vi "Dashboard Main.vi"() -> ()   [LabVIEW 2016]
uses:
  <vilib>/Utility/miscctls.llb/LVRowAndColumnTypeDef.ctl
  <vilib>/event_ctls.llb/eventvkey.ctl
  <vilib>/Rock Robotics/Network Tables/NT Read Numeric Array.vi
  <vilib>/Rock Robotics/Network Tables/NT Write Numeric Array.vi
  <vilib>/Rock Robotics/WPI/Dashboard/WPI_DashboardLogging Global.vi
panel:
  in  "Camera Settings Right":T1={"Frame Rate"=30, "Compression"=30, "Size"=1, "DB Camera Config"=FALSE} {"Frame Rate" scale=1.0..30.0; "Compression" scale=100.0..-1.0; "Size" items=["640x480", "320x240", "160x120"]}
  in  "Camera Name Right":string(combo)="No Camera Selection"
  out "Camera Info":cluster{"Mbps LED":bool, "Mbps":dbl, "fps":dbl} {"fps" format="%#.1g"; "Mbps" format="%#.1g"}
  in  "Camera Settings":T1={"Frame Rate"=30, "Compression"=30, "Size"=1, "DB Camera Config"=FALSE} {"Frame Rate" scale=1.0..30.0; "Compression" scale=100.0..-1.0; "Size" items=["640x480", "320x240", "160x120"]}
  in  "TCP":refnum<k5>
  in  "Rec Mode":enum32{"Stop", "Record", "Playback"}(radio)
  out "Robot IP":string
  out "Image Message":string="Timeout in Camera Communications"
  in  "Dashboard Tab":T2(tab)
  in  "Select Auto":string(combo)="Select Autonomous ..."
  out "NT Connection":bool
  out "MotorChart R":cluster{"Numeric":dbl, "Numeric":dbl}(graph)
  out "MotorChart L":cluster{"Numeric":dbl, "Numeric":dbl}(graph)
  out "MotorSliders R":cluster{"MotorSlide1":dbl, "MotorSlide2":dbl} {"MotorSlide2" scale=-1.0..1.0 scale format="%#_2e"; "MotorSlide1" scale=-1.0..1.0 scale format="%#_2e"}
  out "MotorSliders L":cluster{"MotorSlide1":dbl, "MotorSlide2":dbl} {"MotorSlide2" scale=-1.0..1.0 scale format="%#_2e"; "MotorSlide1" scale=-1.0..1.0 scale format="%#_2e"}
  out "Gyro":dbl(knob) scale=0.0..360.0
  out "JS1 Z":dbl(slide) scale=-1.0..1.0 scale format="%#_2e"
  out "JS1 Graph":cluster{"X":dbl, "Y":dbl}[](graph)
  out "JS1 Buttons":T3
  out "JS2 Z":dbl(slide) scale=-1.0..1.0 scale format="%#_2e"
  out "JS2 Graph":cluster{"X":dbl, "Y":dbl}[](graph)
  out "JS2 Buttons":T3
  out "Mode":T4(ring)=enum."Auto Disabled"
  out "Camera Image Right":T5(plugin-control)
  out "Left Encoder":dbl
  out "Right Encoder":dbl
  in  "Save":bool
  in  "Teleop Controls":T6(tab)
  in  "Y Axis":T7
  in  "X Axis":T7
  in  "Forward Trim":T8={"Trim Max"=0.37, "Trim Min"=0.01, "Trim Deadzone"=0.1, "Trim LR"=TRUE}
  in  "Backward Trim":T8={"Trim Max"=0.5, "Trim Min"=0.05, "Trim Deadzone"=0.1, "Trim LR"=FALSE}
  in  "PID Tuning":enum32{"Drive with PID", "Turn by Angle"}(tab)
  in  "Drive with PID":T9={"Max Speed"=0.7, "P/I/D"=[1.0, 0.0, 0.01], "Min Speed"=0.4, "Accel Distance"=64.0}
  in  "Turn By Angle":T10={"P/I/D"=[0.25, 0.001, 0.0], "Turn Speed"=0.55, "Linearity"=0.6}
  in  "Autonomous Distances":T11(tab)
  in  "Station 1 Angle":dbl=60.0
  in  "Station 1":dbl[](array[numeric])=[97.0, 30.0, -30.0, 120.0]
  in  "Station 2":dbl[](array[numeric])=[82.0, -48.0, 48.0, 120.0]
  in  "Station 3 Angle":dbl=-60.0
  in  "Station 3":dbl[](array[numeric])=[96.0, 30.0, -30.0, 120.0]
  in  "Drive Forward":dbl[](array[numeric])=[82.0, 0.0, 0.0, 0.0]
  in  "Gear and B":dbl[](array[numeric])=[82.0, -48.0, 0.0, 0.0]
  in  "Test Slider":dbl(slide) scale=0.0..100.0 scale format="%#_3g"
  in  "On/Off":bool caption="Solenoid"
  in  "Test Name":u16(ring) items=["Select the test to run..."]
  in  "Test Tree":string(tree)
  in  "Motor":cluster{"Value":dbl, "Enable":bool} {"Value" scale=-1.0..1.0 scale format="%#_3g"}
  out "Progress":T12 {"Test Progress" scale=0.0..100.0}
  in  "Rev/Fwd":cluster{"Forward":bool, "Reverse":bool}
  in  "Test Ring":u16(ring) items=["Monochrome", "Color"]
  out "Cmd Status":string
  in  "Execute Command":bool
  in  "Command Params":string[][](table)
  in  "Command Selection":i32(listbox)
  in  "CheckList":i32(listbox)
  out "Tree":string(tree)
  out "Camera Image":T5(plugin-control)
  in  "Camera Name":string(combo)="No Camera Selection"
  out "Background":bool
  # "HW"
  # "HW"
  # "Joysticks"
  # "Drive Motors"
  # "Front"
  # "Right"
  # "Left"
  # "Back"
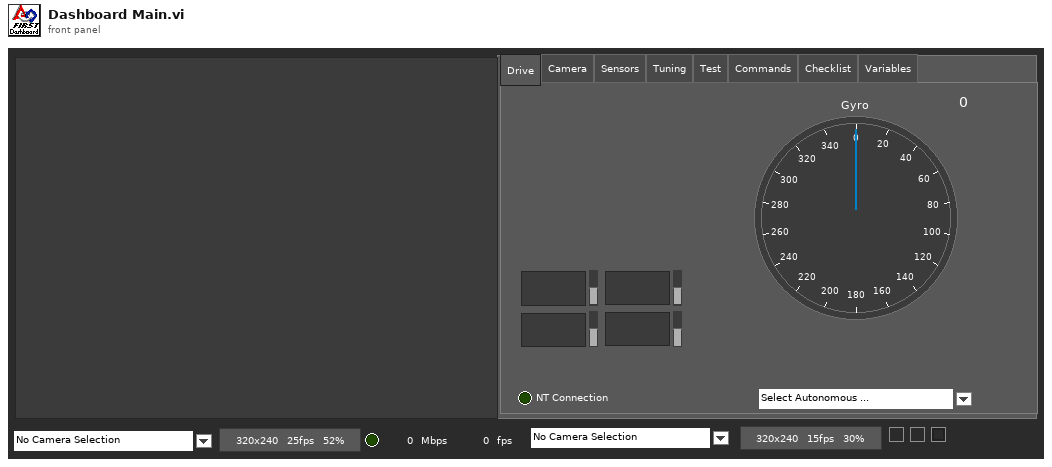
[diagram p1: front panel]
types:
  T1 = cluster{"Frame Rate":i32, "Compression":i32, "Size":u16, "DB Camera Config":bool}
  T2 = enum32{"Drive", "Camera", "Sensors", "Tuning", "Test", "Commands", "Checklist", "Variables"}
  T3 = cluster{bool, bool, bool, bool, bool, bool, bool, bool, bool, bool, bool, bool}
  T4 = enum8{"Tele-Op Disabled", "Tele-Op Enabled", "Auto Disabled", "Auto Enabled", "Test Disabled", "Test Enabled", "Disconnected", "No Code", "E-Stop"}
  T5 = typedef "IMAQ Image.ctl" = refnum<image>
  T6 = enum32{"Speed Sensitivity", "Turn Sensitivity", "Forward Trim", "Backwards Trim"}
  T7 = cluster{"Max Speed":dbl, "Min Speed":dbl, "Deadzone":dbl}
  T8 = cluster{"Trim Max":dbl, "Trim Min":dbl, "Trim Deadzone":dbl, "Trim LR":bool}
  T9 = cluster{"Max Speed":dbl, "P/I/D":dbl[], "Min Speed":dbl, "Accel Distance":dbl}
  T10 = cluster{"P/I/D":dbl[], "Turn Speed":dbl, "Linearity":dbl}
  T11 = enum32{"Station 1", "Station 2", "Station 3", "Drive Forward", "Gear and Back"}
  T12 = cluster{"Test Progress":u8, "Test Progress Text":string}
  T13 = typedef "Image Type" = u32
  T14 = cluster{"IDs":cluster{"RPC field ID":u16, "Unique ID":u16}, "String":string}
  T15 = enum32{"Drive", "Basic", "Custom", "Test", "Checklist", "Variables"}
  T16 = cluster{"Error Strings":string, "Disable Counts":cluster{u16, u16}, "Rail Faults":cluster{u16, u16, u16}, "Robot IP":string, "DB Mode":u8, "Event Info":cluster{"Name":string, "Type":u8, "Number":u16, "Replay":u8}}
  T17 = cluster{"Storage":cluster{"Disk Free":u64, "RAM Block":u32, "RAM free":u32}, "CPU Utilization":cluster{"CPU % ISR":sgl, "CPU % Time Crit":sgl, "CPU % Timed Str":sgl, "CPU % High":sgl, "CPU % Above":sgl, "CPU % Normal":sgl, "CPU % Low":sgl}, "CAN":cluster{"% Bus Utilization":sgl, "Bus Off Cnt":u32, "TX_FIFO Full Cnt":u32, "Receive Error Cnt":u8, "Transmit Error Cnt":u8}, "HID":cluster{"HID Outputs":u32, "Rumble Low":u16, "Rumble High":u16}[]}
  T18 = cluster{"Status bits":cluster{"Test Mode":bool, "Autonomous":bool, "Enabled":bool, "Code Start":bool, "Brownout":bool, "Reserved 2":bool, "Reserved 3":bool, "E-Stop":bool}, "Code Trace":cluster{"Disabled":bool, "TeleOp":bool, "Auto":bool, "Test":bool}, "Controller Type":enum16{"unknown", "cRIO", "roboRio"}, "Code?":enum16{"unknown", "noCode", "code"}, "Battery V":dbl}
  T19 = cluster{"Control Bits":cluster{"TestMode":bool, "Autonomous":bool, "Enabled":bool, "FMS Present":bool, bool, bool, bool, "E-Stop":bool}, "Team Station ":u8, "Countdown":sgl, "Joystick Values":cluster{"Axes":dbl[], "Buttons":bool[], "POVs":i16[]}[]}
  T20 = cluster{"Axes":dbl[], "Buttons":bool[], "POVs":i16[]}[]
  T21 = cluster{"Axes":dbl[], "Buttons":bool[], "POVs":i16[]}
  T22 = cluster{"Buttons[0]":bool, "Buttons[1]":bool, "Buttons[2]":bool, "Buttons[3]":bool, "Buttons[4]":bool, "Buttons[5]":bool, "Buttons[6]":bool, "Buttons[7]":bool, "Buttons[8]":bool, "Buttons[9]":bool, "Buttons[10]":bool, "Buttons[11]":bool}
  T23 = cluster{"X Axis":cluster{"Max Speed":dbl, "Min Speed":dbl, "Deadzone":dbl}, "Y Axis":cluster{"Max Speed":dbl, "Min Speed":dbl, "Deadzone":dbl}, "Forward Trim":cluster{"Trim Max":dbl, "Trim Min":dbl, "Trim Deadzone":dbl, "Trim LR":bool}, "Backward Trim":cluster{"Trim Max":dbl, "Trim Min":dbl, "Trim Deadzone":dbl, "Trim LR":bool}, "Drive with PID":cluster{"Max Speed":dbl, "P/I/D":dbl[], "Min Speed":dbl, "Accel Distance":dbl}, "Turn By Angle":cluster{"P/I/D":dbl[], "Turn Speed":dbl, "Linearity":dbl}}
  T24 = cluster{"Camera Image":refnum<vi>, "Dashboard Tab":refnum<vi>, "Background":refnum<vi>, "Rec Mode":refnum<vi>, "Test Slider":refnum<vi>, "On/Off ":refnum<vi>, "Test Ring":refnum<vi>, "Rev/Fwd":refnum<vi>, "Test Name":refnum<vi>, "Motor":refnum<vi>, "Progress":refnum<vi>, "CheckList":refnum<vi>, "Tree":refnum<vi>, "Test Tree":refnum<vi>, "Command Params":refnum<vi>, "Command Selection":refnum<vi>, "Execute Command":refnum<vi>, "Cmd Status":refnum<vi>, "Camera Settings":refnum<vi>, "Camera Name":refnum<vi>, "Camera Info":refnum<vi>, "Camera Settings Right":refnum<vi>, "Camera Name Right":refnum<vi>, "Camera Image Right":refnum<vi>}
  T25 = cluster{"Operation":enum16{"Update", "Clear"}, "Color Box":u32}[]
  T26 = typedef "eventvkey.ctl" = enum16{"ASCII", "Enter", "Return", "Shift", "Ctrl", "Alt", "Cmd", "Opt", "Caps", "NumLock", "Clear", "Break", "Up", "Down", "Left", "Right", "Insert", "Delete", "Home", "End", "PageUp", "PageDown", "Escape", "Help", "Pause", "ScrollLock", "F1", "F2", "F3", "F4", "F5", "F6", "F7", "F8", "F9", "F10", "F11", "F12", "F13", "F14", "F15", "F16", "F17", "F18", "F19", "F20", "F21", "F22", "F23", "F24", "Play", "VolumeUp", "VolumeDown", "Mute", "Two Byte Char"}
  T27 = cluster{"Image Size":bool, "Image Type":bool, "Pixel Value":bool, "ROI Information":bool, "Zoom Factor":bool}
  T28 = cluster{"Operation":enum16{"Update", "Clear"}, "Color Box":u32}
  T29 = typedef "LVRowAndColumnTypeDef.ctl" = cluster{"Row":i32, "Column":i32}
  T30 = cluster{"Shift":bool, "Ctrl":bool, "Alt":bool, "Cmd":bool, "Opt":bool}
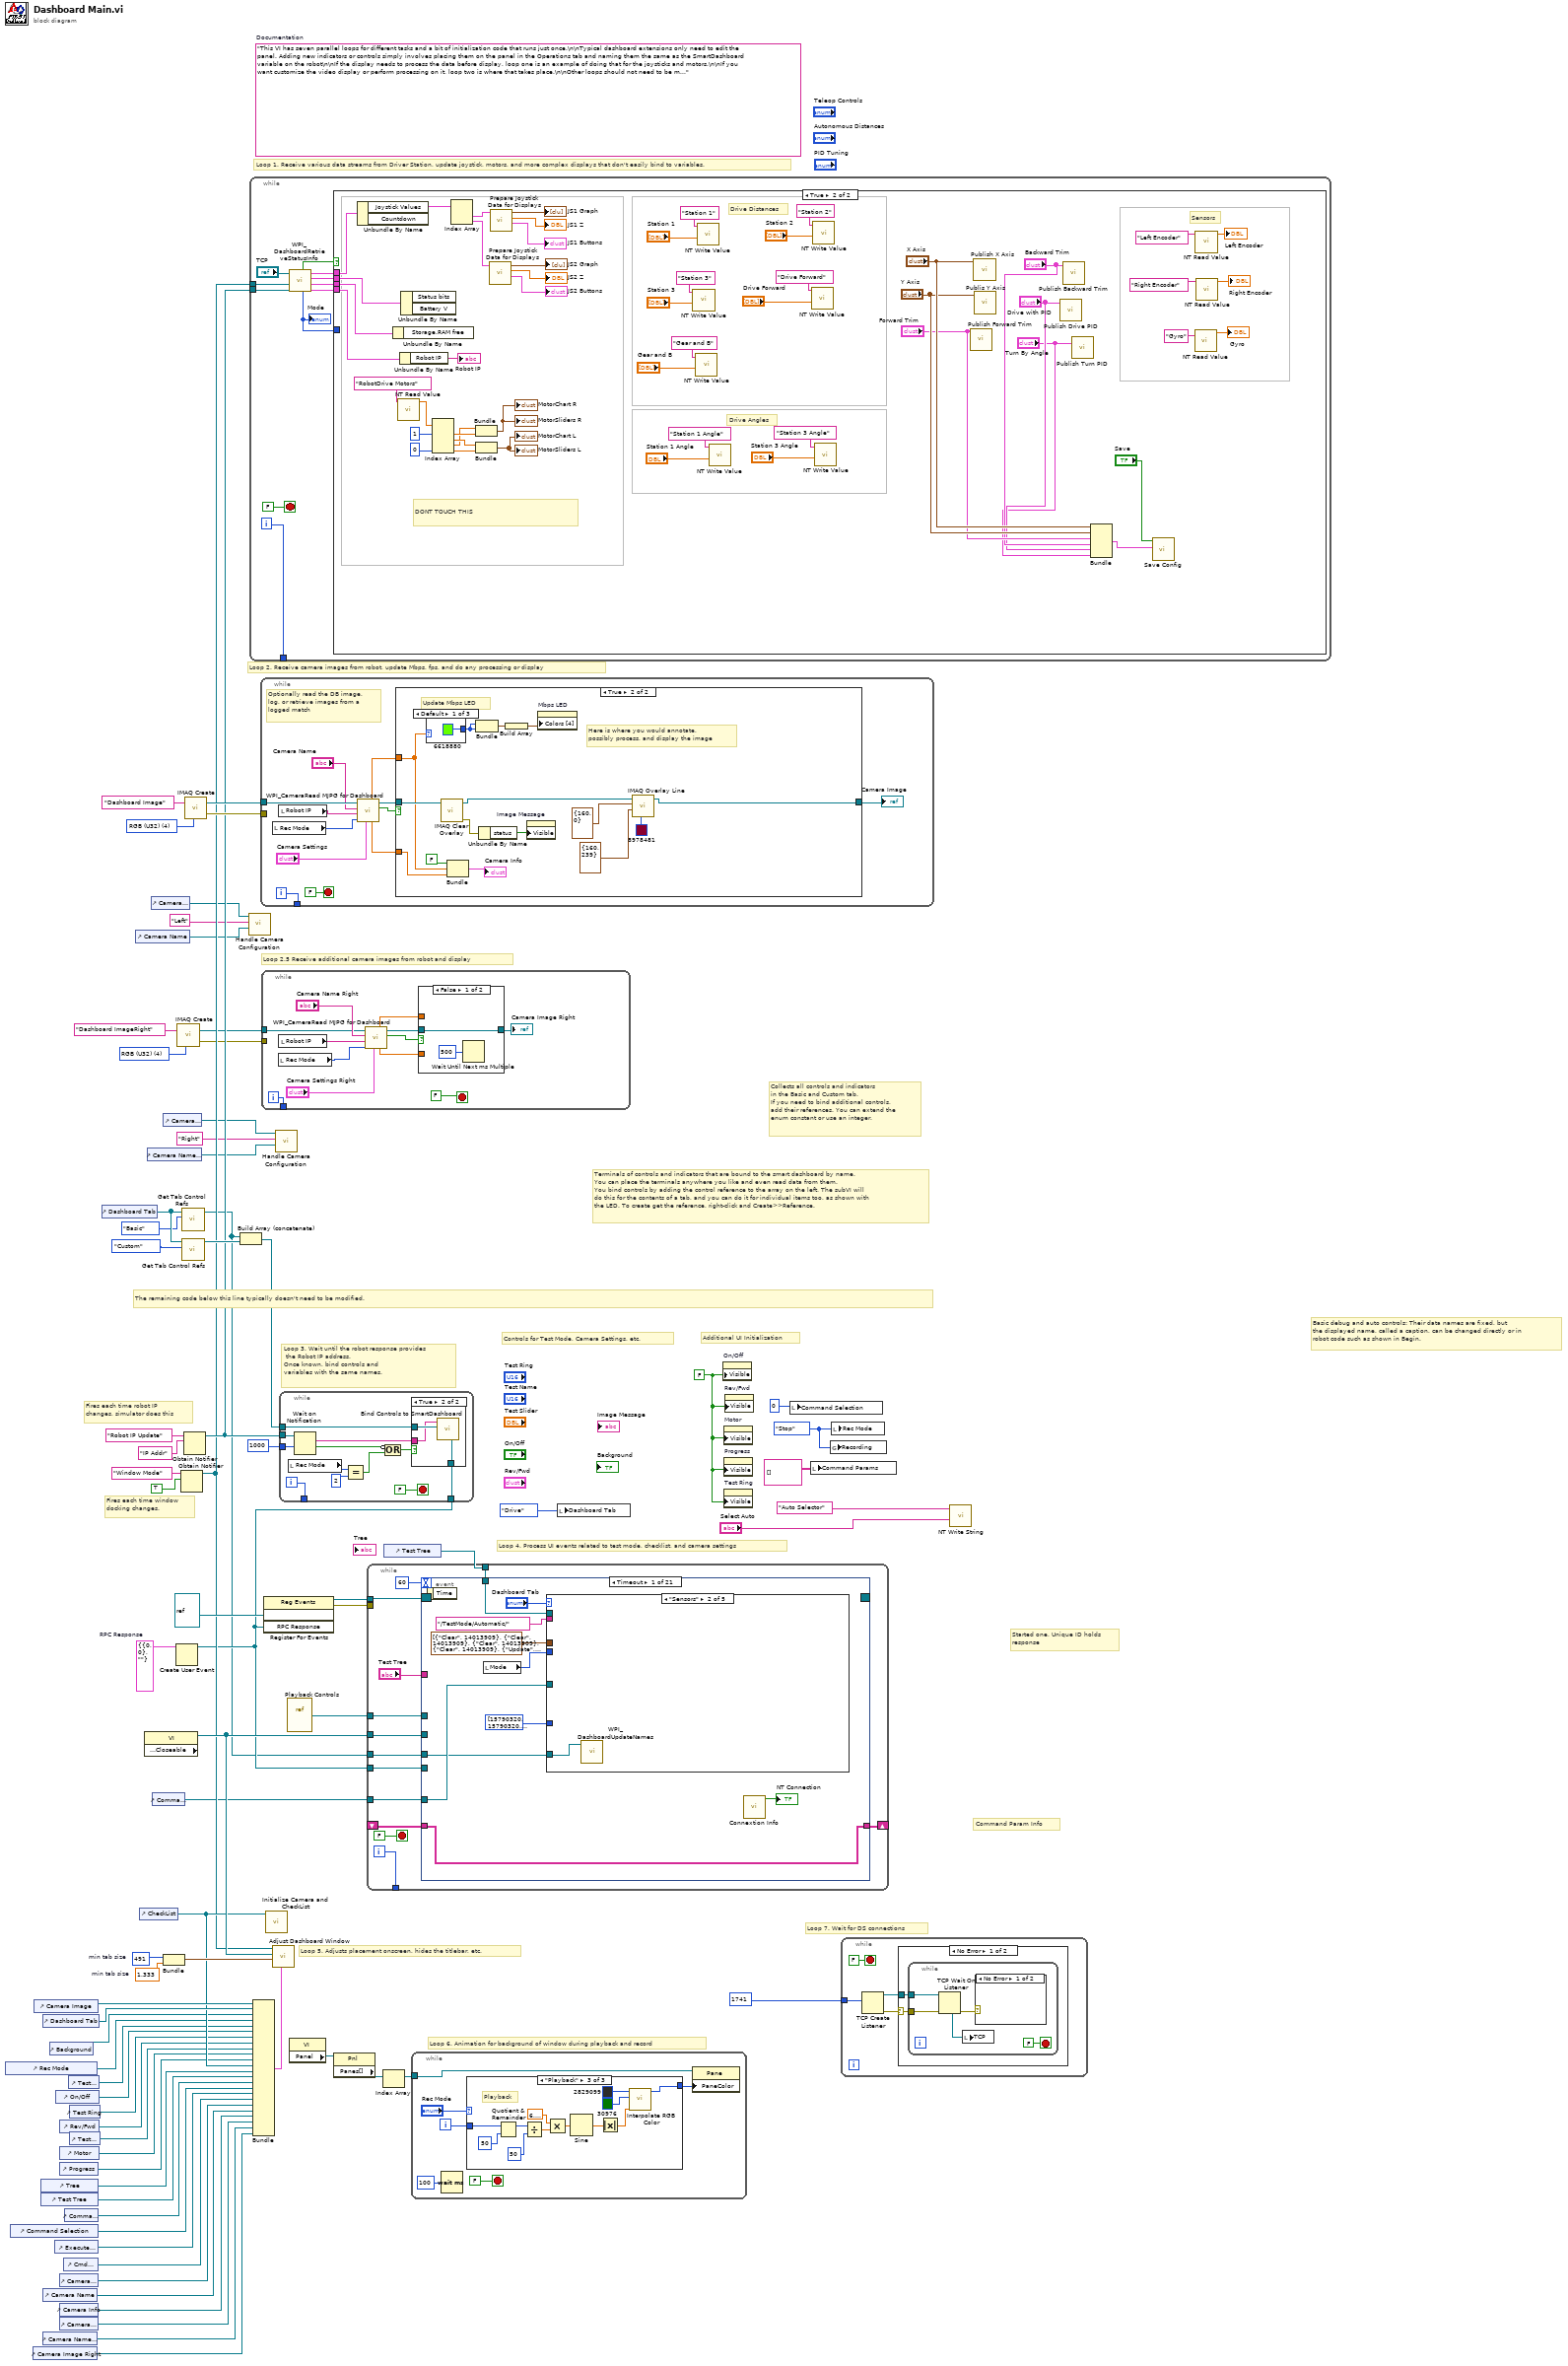
[diagram p0: block diagram]
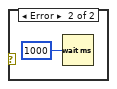
[diagram p3: hidden frame]
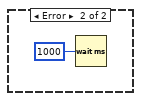
[diagram p4: hidden frame]
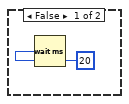
[diagram p5: hidden frame]
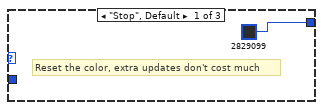
[diagram p6: hidden frame]
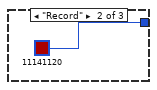
[diagram p7: hidden frame]
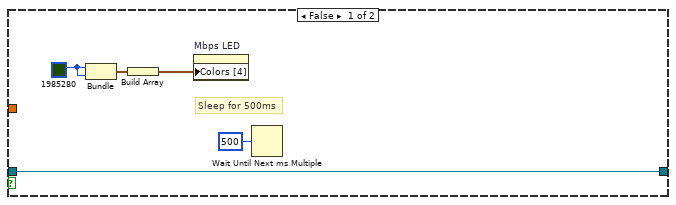
[diagram p9: hidden frame]
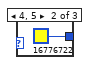
[diagram p10: hidden frame]
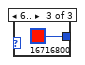
[diagram p11: hidden frame]
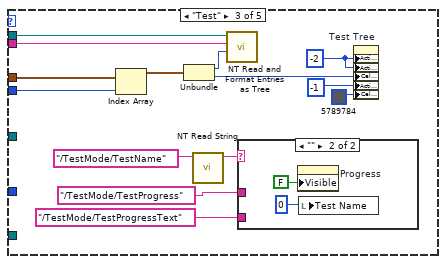
[diagram p13: hidden frame]
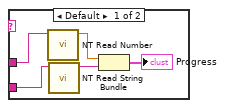
[diagram p14: hidden frame]
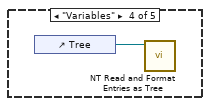
[diagram p15: hidden frame]
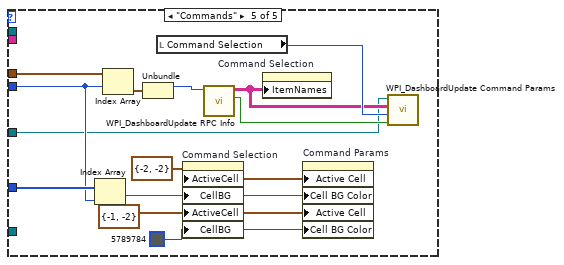
[diagram p16: hidden frame]
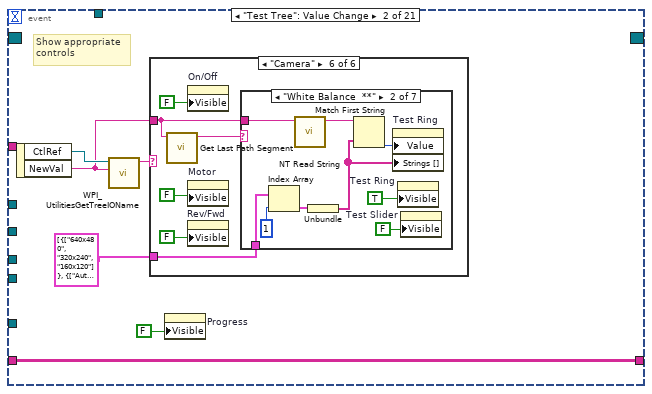
[diagram p17: hidden frame]
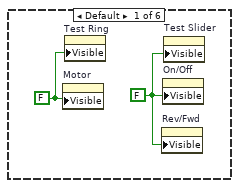
[diagram p18: hidden frame]
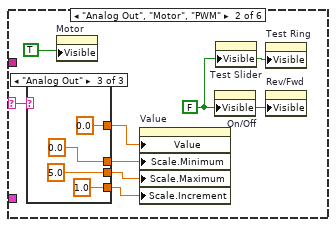
[diagram p19: hidden frame]
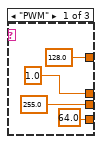
[diagram p20: hidden frame]
diagram:
  w11 = T13 4 items=["Grayscale (U8)", "Grayscale (I16)", "Grayscale (SGL)", "Complex (CSG)", "RGB (U32)", "HSL (U32)", "RGB (U64)"] ("Image Type")
  w27 = T14 {"IDs"={"RPC field ID"=0, "Unique ID"=0}, "String"=""}  # RPC Response
  w51 = 491  # min tab size
  w50 = 1.333  # min tab size
  w58 = enum32{"Stop", "Record", "Playback"}."Stop" ("Rec Mode")
  w34 = FALSE ("Visible")
  (unwired) "This VI has seven parallel loops for different tasks and a bit of initialization code that runs just once.\n\nTypical dashboard extensions only need to edit the panel. Adding new indicators or controls simply involves placing them on the panel in the Operations tab and naming them the same as the SmartDashboard variable on the robot\n\nIf the display needs to process the data before display, loop one is an example of doing that for the joysticks and motors.\n\nIf you want customize the video display or perform processing on it, loop two is where that takes place.\n\nOther loops should not need to be modified. They are pretty standard, and document the task they perform."  # Documentation
  w75 = T13 4 items=["Grayscale (U8)", "Grayscale (I16)", "Grayscale (SGL)", "Complex (CSG)", "RGB (U32)", "HSL (U32)", "RGB (U64)"] ("Image Type")
  # "Loop 2.5 Receive additional camera images from robot and display"
  # "Command Param Info"
  # "Started one, Unique ID holds\nresponse"
  # "Loop 7. Wait for DS connections"
  # "Basic debug and auto controls: Their data names are fixed, but\nthe displayed name, called a caption, can be changed directly or in\nrobot code such as shown in Begin."
  # "Controls for Test Mode, Camera Settings, etc."
  # "Additional UI Initialization"
  # "Loop 6. Animation for background of window during playback and record"
  # "Fires each time robot IP\nchanges, simulator does this"
  # "Fires each time window\ndocking changes."
  # "Collects all controls and indicators\nin the Basic and Custom tab.\nIf you need to bind additional controls,\nadd their references. You can extend the\nenum constant or use an integer."
  # "The remaining code below this line typically doesn't need to be modified."
  # "Loop 4. Process UI events related to test mode, checklist, and camera settings"
  # "Terminals of controls and indicators that are bound to the smart dashboard by name.\nYou can place the terminals anywhere you like and even read data from them.\nYou bind controls by adding the control reference to the array on the left. The subVI will\ndo this for the contents of a tab, and you can do it for individual items too, as shown with\nthe LED. To create get the reference, right-click and Create>>Reference."
  # "Loop 3. Wait until the robot response provides\n the Robot IP address.\nOnce known, bind controls and\nvariables with the same names."
  # "Loop 5. Adjusts placement onscreen, hides the titlebar, etc."
  # "Loop 1. Receive various data streams from Driver Station, update joystick, motors, and more complex displays that don't easily bind to variables."
  # "Loop 2. Receive camera images from robot, update Mbps, fps, and do any processing or display"
  n1 = control-ref of="Rec Mode"() -> (w40:refnum<vi>)
  n2 = control-ref of="Command Selection"() -> (w26:refnum<vi>)
  n3 = control-ref of="Camera Image Right"() -> (w2:refnum<vi>)
  n4 = control-ref of="Camera Image"() -> (w53:refnum<vi>)
  n5 = control-ref of="Tree"() -> (w44:refnum<vi>)
  n6 = control-ref of="Test Tree"() -> (w43:refnum<vi>)
  n7 = control-ref of="Dashboard Tab"() -> (w52:refnum<vi>)
  n8 = control-ref of="Camera Name"() -> (w17:refnum<vi>)
  n9 = control-ref of="Camera Name Right"() -> (w3:refnum<vi>)
  n10 = control-ref of="Background"() -> (w1:refnum<vi>)
  n11 = control-ref of="Execute Command"() -> (w28:refnum<vi>)
  n12 = control-ref of="On/Off"() -> (w38:refnum<vi>)
  n13 = control-ref of="Progress"() -> (w35:refnum<vi>)
  n14 = control-ref of="Camera Settings"() -> (w18:refnum<vi>)
  n15 = control-ref of="Camera Info"() -> (w16:refnum<vi>)
  n16 = control-ref of="Camera Settings Right"() -> (w4:refnum<vi>)
  n17 = control-ref of="Rev/Fwd"() -> (w36:refnum<vi>)
  n18 = control-ref of="Motor"() -> (w41:refnum<vi>)
  n19 = control-ref of="Cmd Status"() -> (w22:refnum<vi>)
  n20 = control-ref of="Command Params"() -> (w29:refnum<vi>)
  n21 = control-ref of="Test Slider"() -> (w39:refnum<vi>)
  n22 = control-ref of="Test Ring"() -> (w37:refnum<vi>)
  n23 = control-ref of="Test Name"() -> (w42:refnum<vi>)
  n24 = control-ref of="Dashboard Tab"() -> (w56:refnum<vi>)
  n25 = control-ref of="Camera Name"() -> (w19:refnum<vi>)
  n26 = control-ref of="CheckList"() -> (w45:refnum<vi>)
  n27 = property class="VI" props=["Front Panel.Closeable"]() -> (reference out=w57:refnum<vi>)  [unwired: 2 in, 2 out]
  n28 = control-ref of="Camera Name Right"() -> (w7:refnum<vi>)
  n29 = control-ref of="Camera Settings"() -> (w20:refnum<vi>)
  n30 = control-ref of="Command Params"() -> (w21:refnum<vi>)
  n31 = control-ref of="Camera Settings Right"() -> (w8:refnum<vi>)
  n32 = Bundle("min tab size"=w51, "min tab size"=w50) -> (w49:cluster{"min tab size":i32, "min tab size":dbl})  [unwired: 1 in]
  n33 = Create User Event(user event datatype=w27) -> (user event=w23:refnum<user-event>)  [unwired: 1 in, 1 out]
  n34 = call "IMAQ Create"("Image Name"="Dashboard ImageRight", "Image Type"=w11) -> ("New Image"=w10:T5, "error out"=w9:errorcluster)  [unwired: 2 in, 1 out]
  n35 = Obtain Notifier(name (unnamed)="Window Mode", notification data type=TRUE) -> (notifier out=w32:refnum<notifier>)  [unwired: 2 in, 2 out]
  n36 = call <vilib>:"Get Tab Control Refs.vi"("Page Index"=T15."Basic" ("Dashboard Tab"), "TabControl in"=w56) -> ("ControlsOnPage"=w15:refnum<vi>[])  [unwired: 9 in]
  n37 = call <vilib>:"Get Tab Control Refs.vi"("Page Index"=T15."Custom" ("Dashboard Tab"), "TabControl in"=w56) -> ("ControlsOnPage"=w55:refnum<vi>[])  [unwired: 9 in]
  n38 = Obtain Notifier(name (unnamed)="Robot IP Update", notification data type="IP Addr" ("name (unnamed)")) -> (notifier out=w33:refnum<notifier>)  [unwired: 2 in, 2 out]
  n39 = call "IMAQ Create"("Image Name"="Dashboard Image", "Image Type"=w75) -> ("New Image"=w73:T5, "error out"=w72:errorcluster)  [unwired: 2 in, 1 out]
  n40 = Build Array (concatenate)(w15, w55) -> (w54:refnum<vi>[])
  n41 = call "Handle Camera Configuration.vi"("CameraNameRef"=w19, "Camera File Name"="Left", "ClusterRef"=w20) -> ()  [unwired: 9 in]
  n42 = while {
    tunnel: [w85] -> _
    tunnel: w33 -> [w79]
    tunnel: w32 -> [w76]
    i -> [w85]
    stop <- FALSE stop-if-true
    n43 = call <vilib>:"WPI_DashboardRetrieveStatusInfo.vi"("Binding Refnum"=w79, "Window Mode Notifier"=w76, "TCP Cnx"="TCP") -> ("Power and Errors"=w80:T16, "Robot Metrics"=w83:T17, "Status Info"=w84:T18, "Control Info"=w81:T19, "Robot Mode"=w78:T4, "Process?"=w82:bool)  [unwired: 3 in]
    "Mode" <- w78
    n44 = case shown="True" w82 {
      tunnel: w84 -> [_ w139]
      tunnel: w83 -> [_ w138]
      tunnel: w81 -> [_ w137]
      tunnel: w80 -> [_ w136]
      tunnel: w78 -> [_ _]
      frame False {
        n45 = Wait (ms)(milliseconds to wait=u32 20) -> ()  [unwired: 1 out]
      }
      frame True {
        # "Drive Angles"
        # "Sensors"
        # "Drive Distances"
        # "DONT TOUCH THIS"
        n46 = Unbundle By Name(w137) -> ("Joystick Values"=w127:T20)  [unwired: 1 out]
        n47 = Unbundle By Name(w138) -> ()  [unwired: 1 out]
        n48 = call-poly <vilib>:"NT Read Value.vi"("Name"="RobotDrive Motors") -> ("Numeric Array"=w117:dbl[])  [unwired: 9 in, 1 out]
        n49 = Unbundle By Name(w136) -> ("Robot IP"=→"Robot IP":string)
        n50 = Unbundle By Name(w139) -> ()  [unwired: 2 out]
        n51 = Index Array(array=w117, index #1=1, index #4=0) -> (element #1=w131:dbl, element #2=w132:dbl, element #3=w130:dbl, element #4=w135:dbl)  [unwired: 2 in]
        n52 = Index Array(array=w127) -> (element #1=w126:T21, element #2=w122:T21)  [unwired: 2 in]
        n53 = Bundle("Numeric"=w130, "Numeric"=w131) -> (→"MotorChart R" →"MotorSliders R":cluster{"Numeric":dbl, "Numeric":dbl})  [unwired: 1 in]
        n54 = Bundle("Numeric"=w132, "Numeric"=w135) -> (→"MotorChart L" →"MotorSliders L":cluster{"Numeric":dbl, "Numeric":dbl})  [unwired: 1 in]
        n55 = call "Prepare Joystick Data for Displays.vi"("Joystick Values"=w122) -> ("Buttons"=→"JS2 Buttons":T22, "Z Axis"=→"JS2 Z":dbl, "Cartesian Data"=→"JS2 Graph":cluster{"X axis":dbl, "X axis":dbl}[])  [unwired: 8 in]
        n56 = call "Prepare Joystick Data for Displays.vi"("Joystick Values"=w126) -> ("Buttons"=→"JS1 Buttons":T22, "Z Axis"=→"JS1 Z":dbl, "Cartesian Data"=→"JS1 Graph":cluster{"X axis":dbl, "X axis":dbl}[])  [unwired: 8 in]
        n57 = call-poly <vilib>:"NT Write Value.vi"("Numeric Array"="Station 3", "Name"="Station 3") -> ()  [unwired: 9 in, 1 out]
        n58 = call-poly <vilib>:"NT Write Value.vi"("Numeric Array"="Gear and B", "Name"="Gear and B") -> ()  [unwired: 9 in, 1 out]
        n59 = call-poly <vilib>:"NT Write Value.vi"("Numeric Array"="Station 1", "Name"="Station 1") -> ()  [unwired: 9 in, 1 out]
        n60 = call-poly <vilib>:"NT Write Value.vi"("Numeric"="Station 1 Angle", "Name"="Station 1 Angle") -> ()  [unwired: 9 in, 1 out]
        n61 = call-poly <vilib>:"NT Write Value.vi"("Numeric Array"="Drive Forward", "Name"="Drive Forward") -> ()  [unwired: 9 in, 1 out]
        n62 = call-poly <vilib>:"NT Write Value.vi"("Numeric Array"="Station 2", "Name"="Station 2") -> ()  [unwired: 9 in, 1 out]
        n63 = call-poly <vilib>:"NT Write Value.vi"("Numeric"="Station 3 Angle", "Name"="Station 3 Angle") -> ()  [unwired: 9 in, 1 out]
        n64 = call "Publish Forward Trim.vi"("Forward Trim"="Forward Trim") -> ()  [unwired: 11 in]
        n65 = call "Publish X Axis.vi"("X Axis"="X Axis") -> ()  [unwired: 11 in]
        n66 = call "Publis Y Axis.vi"("Y Axis"="Y Axis") -> ()  [unwired: 11 in]
        n67 = call "Publish Drive PID.vi"("Drive with PID"="Drive with PID") -> ()  [unwired: 11 in]
        n68 = call "Publish Backward Trim.vi"("Backward Trim"="Backward Trim") -> ()  [unwired: 11 in]
        n69 = call "Publish Turn PID.vi"("Turn By Angle"="Turn By Angle") -> ()  [unwired: 11 in]
        n70 = Bundle("X Axis"="X Axis", "Y Axis"="Y Axis", "Forward Trim"="Forward Trim", "Backward Trim"="Backward Trim", "Drive with PID"="Drive with PID", "Turn By Angle"="Turn By Angle") -> (w89:T23)  [unwired: 1 in]
        n71 = call "Save Config.vi"("Cluster"=w89, "Process"="Save") -> ()  [unwired: 10 in]
        n72 = call-poly <vilib>:"NT Read Value.vi"("Name"="Gyro") -> ("Numeric"=→"Gyro":dbl)  [unwired: 9 in, 1 out]
        n73 = call-poly <vilib>:"NT Read Value.vi"("Name"="Left Encoder") -> ("Numeric"=→"Left Encoder":dbl)  [unwired: 9 in, 1 out]
        n74 = call-poly <vilib>:"NT Read Value.vi"("Name"="Right Encoder") -> ("Numeric"=→"Right Encoder":dbl)  [unwired: 9 in, 1 out]
      }
    }
  }
  n75 = Bundle("Camera Image"=w53, "Dashboard Tab"=w52, "Background"=w1, "Rec Mode"=w40, "Test Slider"=w39, "On/Off"=w38, "Test Ring"=w37, "Rev/Fwd"=w36, "Test Name"=w42, "Motor"=w41, "Progress"=w35, "CheckList"=w45, "Tree"=w44, "Test Tree"=w43, "Command Params"=w29, "Command Selection"=w26, "Execute Command"=w28, "Cmd Status"=w22, "Camera Settings"=w18, "Camera Name"=w17, "Camera Info"=w16, "Camera Settings Right"=w4, "Camera Name Right"=w3, "Camera Image Right"=w2) -> (w46:T24)  [unwired: 1 in]
  n76 = while {
    tunnel: w73 -> [w149]
    tunnel: w72 -> [_]
    tunnel: [w150] -> _
    i -> [w150]
    stop <- FALSE stop-if-true
    # "Optionally read the DB image,\nlog, or retrieve images from a\nlogged match"
    n77 = local read "Rec Mode"() -> (w145:enum32{"Stop", "Record", "Playback"})
    n78 = local read "Robot IP"() -> (w144:string)
    n79 = call <vilib>:"WPI_CameraRead MJPG for Dashboard.vi"("Camera Settings"="Camera Settings", "Rec Mode"=w145, "Robot IP"=w144, "Camera Name"="Camera Name", "Refnum in"=w149) -> ("Active"=w147:bool, "Refnum out"=w148:T5, "FPS"=w146:dbl, "Bandwidth (Mbps)"=w143:dbl)  [unwired: 3 in]
    n80 = case shown="True" w147 {
      tunnel: w148 -> [w152 w167]
      tunnel: w143 -> [_ w164]
      tunnel: w146 -> [_ w165]
      tunnel: [w152 w160] -> w140
      frame False {
        w154 = u32 1985280 ("Color Box")
        # "Sleep for 500ms"
        n81 = Bundle("Color Box"=w154, "Color Box"=w154) -> (w155:cluster{"Color Box":u32, "Color Box":u32})  [unwired: 1 out]
        n82 = Build Array(w155) -> (w153:cluster{"Color Box":u32, "Color Box":u32}[])
        n83 = property on="Mbps LED" class="Bool (strict)"("Colors [4]"=w153) -> ()  [unwired: 2 in, 2 out]
        n84 = Wait Until Next ms Multiple(millisecond multiple=u32 500) -> ()  [unwired: 1 out]
      }
      frame True {
        # "Here is where you would annotate,\npossibly process, and display the image"
        # "Update Mbps LED"
        n85 = case shown="Default" w164 {
          tunnel: [u32 6618880 ("Color Box") u32 16776722 ("Color Box") u32 16716800 ("Color Box")] -> w168
          frame Default {
          }
          frame 4, 5 {
          }
          frame 6.. {
          }
        }
        n86 = call "IMAQ Clear Overlay"("Image"=w167) -> ("error out"=w170:errorcluster, "Image Out"=w161:T5)  [unwired: 2 in, 7 out]
        n87 = Bundle(FALSE, "Bandwidth (Mbps)"=w164, "FPS"=w165) -> (→"Camera Info":cluster{bool, "Bandwidth (Mbps)":dbl, "FPS":dbl})  [unwired: 1 in]
        n88 = Bundle("Color Box"=w168, "Color Box"=w168) -> (w169:cluster{"Color Box":u32, "Color Box":u32})  [unwired: 1 out]
        n89 = Unbundle By Name(w170) -> ("status"=w171:bool)
        n90 = Build Array(w169) -> (w166:cluster{"Color Box":u32, "Color Box":u32}[])
        n91 = property on="Image Message" class="Str"("Visible"=w171) -> ()  [unwired: 2 in, 2 out]
        n92 = property on="Mbps LED" class="Bool (strict)"("Colors [4]"=w166) -> ()  [unwired: 2 in, 2 out]
        n93 = call "IMAQ Overlay Line"("Color"=u32 8978481, "End Point"=cluster{"X":i32, "Y":i32} {"X"=160, "Y"=239}, "Start Point"=cluster{"X":i32, "Y":i32} {"X"=160, "Y"=0}, "Image"=w161) -> ("Image Out"=w160:T5)  [unwired: 6 in, 1 out]
      }
    }
    "Camera Image" <- w140
  }
  n94 = while {
    tunnel: w10 -> [w185]
    tunnel: w9 -> [_]
    tunnel: [w179] -> _
    i -> [w179]
    stop <- FALSE stop-if-true
    n95 = local read "Rec Mode"() -> (w183:enum32{"Stop", "Record", "Playback"})
    n96 = local read "Robot IP"() -> (w184:string)
    n97 = call <vilib>:"WPI_CameraRead MJPG for Dashboard.vi"("Camera Settings"="Camera Settings Right", "Rec Mode"=w183, "Robot IP"=w184, "Camera Name"="Camera Name Right", "Refnum in"=w185) -> ("Active"=w178:bool, "Refnum out"=w181:T5, "FPS"=w176:dbl, "Bandwidth (Mbps)"=w177:dbl)  [unwired: 3 in]
    n98 = case shown="False" w178 {
      tunnel: w181 -> [w187 w189]
      tunnel: w177 -> [_ _]
      tunnel: w176 -> [_ _]
      tunnel: [w187 w189] -> w175
      frame False {
        n99 = Wait Until Next ms Multiple(millisecond multiple=u32 500) -> ()  [unwired: 1 out]
      }
      frame True {
      }
    }
    "Camera Image Right" <- w175
  }
  n100 = register-events(refnum<vi> refnum, w23) -> (reference out=w62:refnum<event-registration>, error out=w61:errorcluster)  [unwired: 2 in]
  n101 = call "Initialize Camera and CheckList.vi"("ListBox in"=w45) -> ()  [unwired: 11 in]
  n102 = call "Adjust Dashboard Window.vi"("Sizing Refnums"=w46, "Size Constraints"=w49, "VI"=w57, "WIn Mode"=w32) -> ()  [unwired: 8 in]
  n103 = call "Handle Camera Configuration.vi"("CameraNameRef"=w7, "Camera File Name"="Right", "ClusterRef"=w8) -> ()  [unwired: 9 in]
  n104 = while {
    tunnel: w54 -> [w201]
    tunnel: w33 -> [w199]
    tunnel: [w197] -> _
    tunnel: u32 1000 ("milliseconds to wait") -> [w196]
    tunnel: w23 -> [w190]
    i -> [w197]
    stop <- FALSE stop-if-true
    n105 = local read "Rec Mode"() -> (w192:enum32{"Stop", "Record", "Playback"})
    n106 = Wait on Notification(notifier=w199, timeout in ms (-1)=w196) -> (notification=w198:string, timed out?=w194:bool)  [unwired: 2 in, 2 out]
    n107 = Equal?(x=w192, y=u16 2 ("Rec Mode")) -> (x = y?=w193:bool)
    n108 = Compound Arithmetic op=OR(invert w194, w193) -> (w195:bool)
    n109 = case shown="True" w195 {
      tunnel: w201 -> [_ w204]
      tunnel: w198 -> [_ w203]
      tunnel: w190 -> [_ w202]
      frame False {
      }
      frame True {
        n110 = call <vilib>:"Bind Controls to SmartDashboard.vi"("RPC ref"=w202, "Bound Control Refs"=w204, "Server IP Address"=w203) -> ()  [unwired: 9 in]
      }
    }
  }
  n111 = vi-ref "Playback Controls.vi"() -> (w63:refnum<vi>)
  n112 = property class="VI"() -> ("Panel"=w65:refnum<vi>)  [unwired: 2 in, 2 out]
  n113 = property class="Pnl"(reference=w65) -> ("Panes[]"=w66:refnum<vi>[])  [unwired: 1 in, 2 out]
  n114 = Index Array(array=w66) -> (element=w64:refnum<vi>)  [unwired: 1 in]
  n115 = control-ref of="Test Tree"() -> (w67:refnum<vi>)
  n116 = while {
    tunnel: [w214] -> _
    tunnel: w67 -> [w213]
    tunnel: w63 -> [w212]
    tunnel: w62 -> [w211]
    tunnel: w61 -> [_]
    tunnel: w57 -> [w210]
    tunnel: w23 -> [w209]
    tunnel: w21 -> [w208]
    shift-right: [w207] -> _
    shift-left: _ -> [w206]
    tunnel: w15 -> [w205]
    i -> [w214]
    stop <- FALSE stop-if-true
    n117 = event shown="[0] Timeout" {
      selector: w211 -> [_ _ _ _ _ _ _ _ _ _ _ _ _ _ _ _ _ _ _ _ _]
      dyn-events: [_ _ _ _ _ _ _ _ _ _ _ _ _ _ _ _ w470 _ _ _ _] -> _
      timeout: u32 60 ("milliseconds to wait") -> [_ _ _ _ _ _ _ _ _ _ _ _ _ _ _ _ _ _ _ _ _]
      tunnel: w213 -> [w226 _ _ _ _ _ _ _ _ _ _ _ _ _ _ _ _ _ _ _ _]
      tunnel: "Test Tree" -> [_ _ _ _ _ _ _ _ _ _ _ w437 w445 w447 w451 w459 _ _ _ _ _]
      tunnel: w212 -> [_ _ _ _ _ _ _ _ _ _ _ _ _ _ _ _ w472 _ w490 _ _]
      tunnel: w210 -> [_ _ _ _ _ _ _ _ _ _ _ _ _ _ _ _ w468 _ _ _ _]
      tunnel: w209 -> [_ _ _ _ _ _ _ _ _ _ _ _ _ _ _ _ w464 _ _ _ _]
      tunnel: w208 -> [w221 _ _ _ _ _ w388 _ _ _ _ _ _ _ _ _ _ _ _ _ _]
      tunnel: [w220 w265 w367 w372 w381 w385 w386 w395 w405 w412 w424 w436 w443 w446 w450 w458 w463 w485 w487 w491 w502] -> w207
      tunnel: w206 -> [w220 w265 w367 w372 w381 w385 w386 _ _ w412 w424 w436 w443 w446 w450 w458 w463 w485 w487 w491 w502]
      tunnel: w205 -> [w218 _ _ _ _ _ _ _ _ _ _ _ _ _ _ _ _ _ _ _ _]
      event Timeout {
        n118 = event-data() -> ()  [unwired: 1 in, 1 out]
        n119 = local read "Mode"() -> (w223:T4)
        n120 = case shown="\"Sensors\"" "Dashboard Tab" {
          tunnel: w226 -> [_ _ w242 _ _]
          tunnel: "/TestMode/Automatic/" ("Name Pattern") -> [_ _ w241 _ _]
          tunnel: T25 [{"Operation"=enum."Clear", "Color Box"=14013909}, {"Operation"=enum."Clear", "Color Box"=14013909}, {"Operation"=enum."Clear", "Color Box"=14013909}, {"Operation"=enum."Clear", "Color Box"=14013909}, {"Operation"=enum."Update", "Color Box"=14013909}, {"Operation"=enum."Update", "Color Box"=16777215}, {"Operation"=enum."Clear", "Color Box"=14013909}, {"Operation"=enum."Clear", "Color Box"=14013909}, {"Operation"=enum."Clear", "Color Box"=14013909}] -> [_ _ w234 _ w258]
          tunnel: w223 -> [_ _ w233 _ w257]
          tunnel: u32[] [15790320, 15790320, 15790320, 15790320, 16777215, 16777215, 15790320, 15790320, 15790320] -> [_ _ _ _ w263]
          tunnel: w221 -> [_ _ _ _ w251]
          tunnel: w218 -> [_ w228 _ _ _]
          frame "Tuning", Default {
          }
          frame "Sensors" {
            n121 = call <vilib>:"WPI_DashboardUpdateNames.vi"("Controls on Tab"=w228) -> ()  [unwired: 11 in]
          }
          frame "Test" {
            w240 = -2 ("Active Item:Row Number")
            n122 = Index Array(array=w234, index=w233) -> (element=w235:T28)
            n123 = Unbundle(w235) -> ("Operation"=w236:enum16{"Update", "Clear"}, "Color Box"=w237:u32)
            n124 = call <vilib>:"NT Read String.vi"("Name"="/TestMode/TestName") -> ("String"=w231:string)  [unwired: 9 in, 1 out]
            n125 = call <vilib>:"NT Read and Format Entries as Tree.vi"("Operation"=w236, "Name Pattern"=w241, "Tree Refnum"=w242) -> ()  [unwired: 7 in, 2 out]
            n126 = case shown="\"\"" w231 {
              tunnel: "/TestMode/TestProgress" ("Name") -> [w244 _]
              tunnel: "/TestMode/TestProgressText" ("Name") -> [w243 _]
              frame Default {
                n127 = call <vilib>:"NT Read Number.vi"("Name"=w244) -> ("Numeric"=w245:dbl)  [unwired: 9 in, 1 out]
                n128 = call <vilib>:"NT Read String.vi"("Name"=w243) -> ("String"=w246:string)  [unwired: 9 in, 1 out]
                n129 = Bundle("Numeric"=w245, "String"=w246) -> (→"Progress":cluster{"Numeric":dbl, "String":string})  [unwired: 1 in]
              }
              frame "" {
                n130 = property on="Progress" class="Clust (strict)"("Visible"=FALSE) -> ()  [unwired: 2 in, 2 out]
                n131 = local write "Test Name"(u16 0) -> ()
              }
            }
            n132 = property on="Test Tree" class="Tree (strict)"("Active Item Row Number"=w240, "ActiveColNum"=w240, "CellBG"=w237, "Active Item Row Number"=-1 ("Active Item:Row Number"), "CellBG"=u32 5789784 ("Color Box")) -> ()  [unwired: 2 in, 2 out]
          }
          frame "Variables" {
            n133 = control-ref of="Tree"() -> (w250:refnum<vi>)
            n134 = call <vilib>:"NT Read and Format Entries as Tree.vi"("Tree Refnum"=w250) -> ()  [unwired: 9 in, 2 out]
          }
          frame "Commands" {
            w259 = u32 5789784 ("Color Box")
            w260 = T29 {"Row"=-1, "Column"=-2} ("Active Cell:Active Cell")
            w262 = T29 {"Row"=-2, "Column"=-2} ("Active Cell:Active Cell")
            n135 = Index Array(array=w263, index=w257) -> (element=w261:u32)
            n136 = Index Array(array=w258, index=w257) -> (element=w256:T28)
            n137 = Unbundle(w256) -> ("Operation"=w255:enum16{"Update", "Clear"})  [unwired: 1 out]
            n138 = local read "Command Selection"() -> (w254:i32)
            n139 = property on="Command Selection" class="MCListbox (strict)"("ActiveCell"=w262, "CellBG"=w261, "ActiveCell"=w260, "CellBG"=w259) -> ()  [unwired: 2 in, 2 out]
            n140 = call <vilib>:"WPI_DashboardUpdate RPC Info.vi"("Operation"=w255) -> ("update"=w253:bool, "commands"=w252:string[][])  [unwired: 9 in]
            n141 = property on="Command Selection" class="MCListbox (strict)"("ItemNames"=w252) -> ()  [unwired: 2 in, 2 out]
            n142 = property on="Command Params" class="Tbl (strict)"("Active Cell"=w262, "Cell BG Color"=w261, "Active Cell"=w260, "Cell BG Color"=w259) -> ()  [unwired: 2 in, 2 out]
            n143 = call <vilib>:"WPI_DashboardUpdate Command Params.vi"("Update"=w253, "NewVal"=w254, "Commands"=w252, "Param Tbl"=w251) -> ()  [unwired: 7 in, 1 out]
          }
        }
        n144 = call <vilib>:"Connextion Info.vi"() -> ("Connected"=→"NT Connection":bool)  [unwired: 10 in, 1 out]
      }
      event "Test Tree": Value Change {
        # "Show appropriate\ncontrols"
        n145 = event-data() -> ("CtlRef"=w268:refnum<vi>, "NewVal"=w266:string)  [unwired: 1 in]
        n146 = call <vilib>:"WPI_UtilitiesGetTreeIOName.vi"("NewVal"=w266, "TreeControl in"=w268) -> ("I/O Name"=w269:string)  [unwired: 9 in]
        n147 = case shown="\"Camera\"" w269 {
          selector: w269 -> [_ w276 _ w298 w307 _]
          tunnel: w266 -> [_ _ w295 w297 _ w314]
          tunnel: cluster{string[]}[] [{["640x480", "320x240", "160x120"]}, {["Auto", "Fixed indoor", "Fixed outdoor 1", "Fixed outdoor 2", "Fixed fluorescent 1", "Fixed fluorescent 2", "Hold current"]}, {["Auto", "Flicker-free 50 Hz", "Flicker-free 60 Hz", "Hold current"]}, {["None", "Prioritize frame rate", "Prioritize image quality"]}, {["Monochrome", "Color"]}] -> [_ _ _ _ _ w313]
          frame Default {
            w271 = FALSE ("Visible")
            w270 = FALSE ("Visible")
            n148 = property on="Motor" class="Clust (strict)"("Visible"=w270) -> ()  [unwired: 2 in, 2 out]
            n149 = property on="Test Ring" class="Ring (strict)"("Visible"=w270) -> ()  [unwired: 2 in, 2 out]
            n150 = property on="Rev/Fwd" class="Clust (strict)"("Visible"=w271) -> ()  [unwired: 2 in, 2 out]
            n151 = property on="On/Off" class="Bool (strict)"("Visible"=w271) -> ()  [unwired: 2 in, 2 out]
            n152 = property on="Test Slider" class="Slide (strict)"("Visible"=w271) -> ()  [unwired: 2 in, 2 out]
          }
          frame "Analog Out", "Motor", "PWM" {
            w277 = FALSE ("Visible")
            n153 = case shown="\"Analog Out\"" w276 {
              tunnel: [1.0 ("Value") -1.0 ("Value") 0.0 ("Value")] -> w275
              tunnel: [255.0 ("Value") 1.0 ("Value") 5.0 ("Value")] -> w274
              tunnel: [128.0 ("Value") 0.0 ("Value") 0.0 ("Value")] -> w273
              tunnel: [64.0 ("Value") 0.5 ("Value") 1.0 ("Value")] -> w272
              frame "PWM" {
              }
              frame "Motor", Default {
              }
              frame "Analog Out" {
              }
            }
            n154 = property on="Motor" class="Clust (strict)"("Visible"=TRUE) -> ()  [unwired: 2 in, 2 out]
            n155 = property on="Value" class="Slide (strict)"("Value"=w273, "Scale.Minimum"=w275, "Scale.Maximum"=w274, "Scale.Increment"=w272) -> ()  [unwired: 2 in, 2 out]
            n156 = property on="On/Off" class="Bool (strict)"("Visible"=w277) -> ()  [unwired: 2 in, 2 out]
            n157 = property on="Test Slider" class="Slide (strict)"("Visible"=w277) -> ()  [unwired: 2 in, 2 out]
            n158 = property on="Test Ring" class="Ring (strict)"("Visible"=w277) -> ()  [unwired: 2 in, 2 out]
            n159 = property on="Rev/Fwd" class="Clust (strict)"("Visible"=w277) -> ()  [unwired: 2 in, 2 out]
          }
          frame "Servo" {
            w293 = FALSE ("Visible")
            n160 = call <vilib>:"NT Read Number.vi"("Name"=w295) -> ("Numeric"=w294:dbl)  [unwired: 9 in, 1 out]
            n161 = property on="Test Slider" class="Slide (strict)"("Visible"=TRUE, "Scale.Maximum"=170.0 ("Scale.Range:Maximum")) -> ()  [unwired: 2 in, 2 out]
            n162 = local write "Test Slider"(w294) -> ()
            n163 = property on="Motor" class="Clust (strict)"("Visible"=w293) -> ()  [unwired: 2 in, 2 out]
            n164 = property on="Rev/Fwd" class="Clust (strict)"("Visible"=w293) -> ()  [unwired: 2 in, 2 out]
            n165 = property on="On/Off" class="Bool (strict)"("Visible"=w293) -> ()  [unwired: 2 in, 2 out]
            n166 = property on="Test Ring" class="Ring (strict)"("Visible"=w293) -> ()  [unwired: 2 in, 2 out]
          }
          frame "Relay", "Solenoid" {
            w296 = FALSE ("Visible")
            n167 = property on="Motor" class="Clust (strict)"("Visible"=w296) -> ()  [unwired: 2 in, 2 out]
            n168 = property on="Test Slider" class="Slide (strict)"("Visible"=w296) -> ()  [unwired: 2 in, 2 out]
            n169 = Search and Replace String(input string=w297, search string="/Value  **", replace string="/Direction") -> (result string=w303:string)  [unwired: 5 in, 3 out]
            n170 = property on="Test Ring" class="Ring (strict)"("Visible"=w296) -> ()  [unwired: 2 in, 2 out]
            n171 = call <vilib>:"NT Read String.vi"("Name"=w303) -> ("String"=w301:string)  [unwired: 9 in, 1 out]
            n172 = Equal?(x="Both directions", y=w301) -> (x = y?=w299:bool)
            n173 = Not(x=w299) -> (.not. x?=w300:bool)
            n174 = property on="Rev/Fwd" class="Clust (strict)"("Visible"=w299) -> ()  [unwired: 2 in, 2 out]
            n175 = property on="On/Off" class="Bool (strict)"("Visible"=w300, "Caption.Text"=w298) -> ()  [unwired: 2 in, 2 out]
          }
          frame "Compressor", "Digital Out" {
            w306 = FALSE ("Visible")
            # "Get direction and finish"
            n176 = property on="Motor" class="Clust (strict)"("Visible"=w306) -> ()  [unwired: 2 in, 2 out]
            n177 = property on="Test Slider" class="Slide (strict)"("Visible"=w306) -> ()  [unwired: 2 in, 2 out]
            n178 = property on="Test Ring" class="Ring (strict)"("Visible"=w306) -> ()  [unwired: 2 in, 2 out]
            n179 = property on="On/Off" class="Bool (strict)"("Visible"=TRUE, "Caption.Text"=w307) -> ()  [unwired: 2 in, 2 out]
            n180 = property on="Rev/Fwd" class="Clust (strict)"("Visible"=FALSE) -> ()  [unwired: 2 in, 2 out]
          }
          frame "Camera" {
            n181 = call <vilib>:"Get Last Path Segment.vi"("String in"=w314) -> ("String out"=w315:string)  [unwired: 10 in]
            n182 = property on="On/Off" class="Bool (strict)"("Visible"=FALSE) -> ()  [unwired: 2 in, 2 out]
            n183 = property on="Motor" class="Clust (strict)"("Visible"=FALSE) -> ()  [unwired: 2 in, 2 out]
            n184 = property on="Rev/Fwd" class="Clust (strict)"("Visible"=FALSE) -> ()  [unwired: 2 in, 2 out]
            n185 = case shown="\"White Balance  **\"" w315 {
              tunnel: w314 -> [w321 w330 w339 w348 w357 _ w363]
              tunnel: w313 -> [w319 w327 w336 w345 w354 _ _]
              frame "Size  **" {
                n186 = Index Array(array=w319) -> (element=w318:cluster{string[]})  [unwired: 1 in]
                n187 = call <vilib>:"NT Read String.vi"("Name"=w321) -> ("String"=w320:string)  [unwired: 9 in, 1 out]
                n188 = Unbundle(w318) -> (w316:string[])
                n189 = Match First String(2:w316, 3:w320) -> (0:w317:i32)  [unwired: 1 out]
                n190 = property on="Test Ring" class="Ring (strict)"("Value"=w317, "Strings []"=w316) -> ()  [unwired: 2 in, 2 out]
                n191 = property on="Test Ring" class="Ring (strict)"("Visible"=TRUE) -> ()  [unwired: 2 in, 2 out]
                n192 = property on="Test Slider" class="Slide (strict)"("Visible"=FALSE) -> ()  [unwired: 2 in, 2 out]
              }
              frame "White Balance  **" {
                n193 = Index Array(array=w327, index=1) -> (element=w328:cluster{string[]})
                n194 = call <vilib>:"NT Read String.vi"("Name"=w330) -> ("String"=w329:string)  [unwired: 9 in, 1 out]
                n195 = Unbundle(w328) -> (w325:string[])
                n196 = Match First String(2:w325, 3:w329) -> (0:w324:i32)  [unwired: 1 out]
                n197 = property on="Test Ring" class="Ring (strict)"("Value"=w324, "Strings []"=w325) -> ()  [unwired: 2 in, 2 out]
                n198 = property on="Test Ring" class="Ring (strict)"("Visible"=TRUE) -> ()  [unwired: 2 in, 2 out]
                n199 = property on="Test Slider" class="Slide (strict)"("Visible"=FALSE) -> ()  [unwired: 2 in, 2 out]
              }
              frame "Exposure  **" {
                n200 = Index Array(array=w336, index=2) -> (element=w337:cluster{string[]})
                n201 = call <vilib>:"NT Read String.vi"("Name"=w339) -> ("String"=w338:string)  [unwired: 9 in, 1 out]
                n202 = Unbundle(w337) -> (w333:string[])
                n203 = Match First String(2:w333, 3:w338) -> (0:w334:i32)  [unwired: 1 out]
                n204 = property on="Test Ring" class="Ring (strict)"("Value"=w334, "Strings []"=w333) -> ()  [unwired: 2 in, 2 out]
                n205 = property on="Test Ring" class="Ring (strict)"("Visible"=TRUE) -> ()  [unwired: 2 in, 2 out]
                n206 = property on="Test Slider" class="Slide (strict)"("Visible"=FALSE) -> ()  [unwired: 2 in, 2 out]
              }
              frame "Exposure Priority  **" {
                n207 = Index Array(array=w345, index=3) -> (element=w346:cluster{string[]})
                n208 = call <vilib>:"NT Read String.vi"("Name"=w348) -> ("String"=w347:string)  [unwired: 9 in, 1 out]
                n209 = Unbundle(w346) -> (w342:string[])
                n210 = Match First String(2:w342, 3:w347) -> (0:w343:i32)  [unwired: 1 out]
                n211 = property on="Test Ring" class="Ring (strict)"("Value"=w343, "Strings []"=w342) -> ()  [unwired: 2 in, 2 out]
                n212 = property on="Test Ring" class="Ring (strict)"("Visible"=TRUE) -> ()  [unwired: 2 in, 2 out]
                n213 = property on="Test Slider" class="Slide (strict)"("Visible"=FALSE) -> ()  [unwired: 2 in, 2 out]
              }
              frame "Color Enable  **" {
                n214 = Index Array(array=w354, index=4) -> (element=w355:cluster{string[]})
                n215 = call <vilib>:"NT Read String.vi"("Name"=w357) -> ("String"=w356:string)  [unwired: 9 in, 1 out]
                n216 = Unbundle(w355) -> (w351:string[])
                n217 = Match First String(2:w351, 3:w356) -> (0:w352:i32)  [unwired: 1 out]
                n218 = property on="Test Ring" class="Ring (strict)"("Value"=w352, "Strings []"=w351) -> ()  [unwired: 2 in, 2 out]
                n219 = property on="Test Ring" class="Ring (strict)"("Visible"=TRUE) -> ()  [unwired: 2 in, 2 out]
                n220 = property on="Test Slider" class="Slide (strict)"("Visible"=FALSE) -> ()  [unwired: 2 in, 2 out]
              }
              frame Default {
                n221 = property on="Test Ring" class="Ring (strict)"("Visible"=FALSE) -> ()  [unwired: 2 in, 2 out]
                n222 = property on="Test Slider" class="Slide (strict)"("Visible"=FALSE) -> ()  [unwired: 2 in, 2 out]
              }
              frame "Brightness  **", "Color Level  **", "Compression  **", "FPS  **", "Sharpness  **" {
                n223 = call <vilib>:"NT Read Number.vi"("Name"=w363) -> ("Numeric"=w362:dbl)  [unwired: 9 in, 1 out]
                n224 = local write "Test Slider"(w362) -> ()
                n225 = property on="Test Slider" class="Slide (strict)"("Visible"=TRUE, "Scale.Maximum"=100.0 ("Scale.Range:Maximum")) -> ()  [unwired: 2 in, 2 out]
                n226 = property on="Test Ring" class="Ring (strict)"("Visible"=FALSE) -> ()  [unwired: 2 in, 2 out]
              }
            }
          }
        }
        n227 = property on="Progress" class="Clust (strict)"("Visible"=FALSE) -> ()  [unwired: 2 in, 2 out]
      }
      event "Test Name": Mouse Enter {
        # "Populate the ring with the list of tests"
        n228 = event-data() -> ()  [unwired: 1 in, 1 out]
        n229 = call <vilib>:"NT Read String Array.vi"("Name"="/TestMode/TestList") -> ("String Array"=w371:string[])  [unwired: 9 in, 1 out]
        n230 = Build Array (concatenate)("Select the test to run...", w371) -> (w370:string[])
        n231 = property on="Test Name" class="Ring (strict)"("Strings []"=w370) -> ()  [unwired: 2 in, 2 out]
      }
      event "Test Name": Value Change {
        w373 = FALSE ("Visible")
        # "Tell the robot the test name to run"
        n232 = event-data() -> ("NewVal"=w377:u16)  [unwired: 1 in]
        n233 = property on="Test Name" class="Ring (strict)"() -> ("Strings []"=w378:string[])  [unwired: 2 in, 2 out]
        n234 = local write "Progress"(T12 {"Test Progress"=0, "Test Progress Text"=""} ("Progress")) -> ()
        n235 = Index Array(array=w378, index=w377) -> (element=w376:string)
        n236 = call <vilib>:"NT Write String.vi"("String"=w376, "Name"="/TestMode/TestName") -> ()  [unwired: 9 in, 1 out]
        n237 = property on="Progress" class="Clust (strict)"("Visible"=TRUE) -> ()  [unwired: 2 in, 2 out]
        n238 = property on="Motor" class="Clust (strict)"("Visible"=w373) -> ()  [unwired: 2 in, 2 out]
        n239 = property on="Test Slider" class="Slide (strict)"("Visible"=w373) -> ()  [unwired: 2 in, 2 out]
        n240 = property on="On/Off" class="Bool (strict)"("Visible"=w373) -> ()  [unwired: 2 in, 2 out]
        n241 = property on="Rev/Fwd" class="Clust (strict)"("Visible"=w373) -> ()  [unwired: 2 in, 2 out]
        n242 = property on="Test Ring" class="Ring (strict)"("Visible"=w373) -> ()  [unwired: 2 in, 2 out]
      }
      event "Select Auto": Mouse Enter {
        # "Populate the combo box with the list of autonomous options"
        n243 = event-data() -> ()  [unwired: 1 in, 1 out]
        n244 = call <vilib>:"NT Read String Array.vi"("Name"="Auto List") -> ("String Array"=w380:string[])  [unwired: 9 in, 1 out]
        n245 = property on="Select Auto" class="CmbBox"("Strings[]"=w380) -> ()  [unwired: 2 in, 2 out]
      }
      event "Select Auto": Value Change {
        # "User modified the Auto Selection. Write to NT variable so robot knows."
        n246 = event-data() -> ("NewVal"=w383:string)  [unwired: 1 in]
        n247 = call <vilib>:"NT Write String.vi"("String"=w383, "Name"="Auto Selector") -> ()  [unwired: 9 in, 1 out]
      }
      event "Command Selection": Value Change {
        # "Get the params and show in table"
        n248 = event-data() -> ("NewVal"=w389:i32)  [unwired: 1 in]
        n249 = property on="Command Selection" class="MCListbox (strict)"() -> ("ItemNames"=w387:string[][])  [unwired: 2 in, 2 out]
        n250 = call <vilib>:"WPI_DashboardUpdate Command Params.vi"("NewVal"=w389, "Commands"=w387, "Param Tbl"=w388) -> ()  [unwired: 8 in, 1 out]
      }
      event "Execute Command": Value Change {
        # "Started one, Unique ID holds\nresponse"
        n251 = event-data() -> ()  [unwired: 1 in, 1 out]
        n252 = property on="Command Selection" class="MCListbox (strict)"() -> ("ItemNames"=w400:string[][])  [unwired: 2 in, 2 out]
        n253 = Index Array(array=w400, index (row)="Command Selection", index (col)=0) -> (element=w398:string)
        n254 = call <vilib>:"Invoke Commands.vi"("Command Params"="Command Params", "Function Name"=w398) -> ("Params"=w394:u8, "Started"=w393:bool)  [unwired: 7 in, 1 out]
        n255 = Array Subset(array="Command Params", length (row)=w394) -> (w395:string[][])  [unwired: 3 in]
        n256 = Select(t="Executing" ("Cmd Status"), s=w393, f="" ("Cmd Status")) -> (s? t:f=→"Cmd Status":string)
      }
      event "Command Selection": Double Click {
        n257 = event-data() -> ("Row"=w408:i32)  [unwired: 1 in]
        n258 = property on="Command Selection" class="MCListbox (strict)"() -> ("ItemNames"=w411:string[][])  [unwired: 2 in, 2 out]
        n259 = local read "Command Params"() -> (w407:string[][])
        n260 = Index Array(array=w411, index (row)=w408, index (col)=0) -> (element=w409:string)
        n261 = call <vilib>:"Invoke Commands.vi"("Command Params"=w407, "Function Name"=w409) -> ("Params"=w406:u8, "Started"=w401:bool)  [unwired: 7 in, 1 out]
        n262 = Array Subset(array=w407, length (row)=w406) -> (w405:string[][])  [unwired: 3 in]
        n263 = Select(t="Executing" ("Cmd Status"), s=w401, f="" ("Cmd Status")) -> (s? t:f=w402:string)
        n264 = local write "Cmd Status"(w402) -> ()
      }
      event "CheckList": Double Click {
        # "Shift clears all"
        # "Update symbols on the listbox"
        n265 = event-data() -> ("PlatMods.Shift"=w413:bool, "Row"=w415:i32)  [unwired: 1 in]
        n266 = case shown="True" w413 {
          tunnel: w415 -> [w419 _]
          tunnel: 1 -> [w418 _]
          frame False {
            n267 = property on="CheckList" class="LstBox (strict)"() -> ("Item Symbols"=w417:i32[])  [unwired: 2 in, 2 out]
            n268 = Replace Array Subset(array=w417, new element=w418, index=w419) -> (w416:i32[])
            n269 = property on="CheckList" class="LstBox (strict)"("Item Symbols"=w416) -> ()  [unwired: 2 in, 2 out]
          }
          frame True {
            w420 = 0 ("Top Row")
            n270 = property on="CheckList" class="LstBox (strict)"() -> ("Number of Rows"=w422:u32)  [unwired: 2 in, 2 out]
            n271 = Initialize Array(0, w422) -> (w421:i32[])
            n272 = property on="CheckList" class="LstBox (strict)"("Top Row"=w420, "Value"=w420, "Item Symbols"=w421) -> ()  [unwired: 2 in, 2 out]
          }
        }
      }
      event "CheckList": Key Down {
        # "Update symbols on the listbox\nLeft and right keys check and uncheck"
        n273 = event-data() -> ("VKey"=w426:T26)  [unwired: 1 in]
        n274 = case shown="\"Left\", \"Right\"" w426 {
          selector: w426 -> [w431 _]
          tunnel: eventvkey."Left" ("VKey") -> [w429 _]
          frame "Left", "Right" {
            n275 = Equal?(x=w429, y=w431) -> (x = y?=w430:bool)
            n276 = Select(t=0, s=w430, f=1) -> (s? t:f=w432:i32)
            n277 = property on="CheckList" class="LstBox (strict)"() -> ("Item Symbols"=w435:i32[])  [unwired: 2 in, 2 out]
            n278 = Replace Array Subset(array=w435, new element=w432, index="CheckList") -> (w434:i32[])
            n279 = property on="CheckList" class="LstBox (strict)"("Item Symbols"=w434) -> ()  [unwired: 2 in, 2 out]
          }
          frame Default {
          }
        }
      }
      event "Motor.Enable": Value Change {
        # "When the test mode otor enable helper is set, update that\ntree row item's value"
        n280 = event-data() -> ("NewVal"=w441:bool)  [unwired: 1 in]
        n281 = Unbundle("Motor") -> ("Value"=w440:dbl)  [unwired: 1 out]
        n282 = Select(t=w440, s=w441, f=0.0) -> (s? t:f=w438:dbl)
        n283 = call <vilib>:"NT Write Number.vi"("Numeric"=w438, "Name"=w437) -> ()  [unwired: 9 in, 1 out]
      }
      event "Test Slider": Value Change {
        # "When the test mode slider helper is set, update that\ntree row item's value"
        n284 = event-data() -> ("NewVal"=w444:dbl)  [unwired: 1 in]
        n285 = call <vilib>:"NT Write Number.vi"("Numeric"=w444, "Name"=w445) -> ()  [unwired: 9 in, 1 out]
      }
      event "On/Off": Value Change {
        # "When the test mode on/off helper value is set, update that\ntree row item's value"
        n286 = event-data() -> ("NewVal"=w449:bool)  [unwired: 1 in]
        n287 = Boolean To (0,1)(Boolean=w449) -> (0, 1=w448:i16)
        n288 = call <vilib>:"NT Write Number.vi"("Numeric"=w448, "Name"=w447) -> ()  [unwired: 9 in, 1 out]
      }
      event "Rev/Fwd": Value Change {
        # "When the test mode helper value for relays is set, update that\ntree row item's value"
        n289 = event-data() -> ("NewVal.Forward"=w457:bool, "NewVal.Reverse"=w456:bool)  [unwired: 1 in]
        n290 = Boolean To (0,1)(Boolean=w457) -> (0, 1=w453:i16)
        n291 = Boolean To (0,1)(Boolean=w456) -> (0, 1=w455:i16)
        n292 = Negate(x=w455) -> (-x=w454:i16)
        n293 = Add(x=w453, y=w454) -> (x+y=w452:i16)
        n294 = call <vilib>:"NT Write Number.vi"("Numeric"=w452, "Name"=w451) -> ()  [unwired: 9 in, 1 out]
      }
      event "Test Ring": Value Change {
        # "When a test mode helper value is selected from the ring,\nset the tree item's variable to the string value"
        n295 = event-data() -> ("NewVal"=w461:u16)  [unwired: 1 in]
        n296 = property on="Test Ring" class="Ring (strict)"() -> ("Strings []"=w462:string[])  [unwired: 2 in, 2 out]
        n297 = Index Array(array=w462, index=w461) -> (element=w460:string)
        n298 = call <vilib>:"NT Write String.vi"("String"=w460, "Name"=w459) -> ()  [unwired: 9 in, 1 out]
      }
      event "Rec Mode": Value Change {
        # "Update globals for recording mode and path to read log from.\nClear when logging and let NetworkTables set path for vision to\nuse."
        n299 = event-data() -> ("NewVal"=w473:enum32{"Stop", "Record", "Playback"})  [unwired: 1 in]
        n300 = global write "WPI_DashboardLogging Global.vi" "Logging Filename"(path "") -> ()
        n301 = global write "WPI_DashboardLogging Global.vi" "Recording"(w473) -> ()
        n302 = case shown="\"Playback\"" w473 {
          tunnel: w472 -> [_ w475 w484]
          tunnel: [_ _ w483] -> w470
          tunnel: [_ _ w482] -> _
          tunnel: w468 -> [_ _ w480]
          tunnel: cluster{i32, i32} {-250, 170} -> [_ _ w479]
          tunnel: [_ _ T27 {"Image Size"=TRUE, "Image Type"=TRUE, "Pixel Value"=TRUE, "ROI Information"=TRUE, "Zoom Factor"=FALSE} ("Image Information Shown:All Elements")] -> w466
          tunnel: [_ _ TRUE ("Zoom Factor")] -> w465
          tunnel: w464 -> [_ _ w476]
          frame Default {
          }
          frame "Stop", "Record" {
            # "Place Window too"
            n303 = invoke class="VI" method="FP.Close"(reference=w475) -> (reference out=w474:refnum<vi>)  [unwired: 2 in, 2 out]
            n304 = invoke class="VI" method="Abort VI"(reference=w474) -> ()  [unwired: 2 in, 3 out]
          }
          frame "Playback" {
            n305 = call "Open Playback Panel.vi"("Offset"=w479, "DB VI Ref"=w480, "Playback in"=w484) -> ("Playback out"=w481:refnum<vi>)  [unwired: 8 in]
            n306 = register-events(w481, w476) -> (reference out=w483:refnum<event-registration>, error out=w482:errorcluster)  [unwired: 2 in]
          }
        }
        n307 = property on="Camera Image" class="ImageControl"("Image Information Shown"=w466, "Image Information Visible"=w465) -> ()  [unwired: 2 in, 2 out]
        n308 = call <vilib>:"WPI_DashboardNT Log FieldName Cache.vi"("Operation"=enum16{"Lookup/Add", "Index", "Clear"}."Clear") -> ()  [unwired: 8 in, 3 out]
      }
      event Panel Close {
        w486 = enum32{"Stop", "Record", "Playback"}."Stop" ("Rec Mode")
        # "Playback window has been closed, abort"
        n309 = event-data() -> ()  [unwired: 1 in, 4 out]
        n310 = local write "Rec Mode"(w486) -> ()
        n311 = global write "WPI_DashboardLogging Global.vi" "Recording"(w486) -> ()
      }
      event Panel Close {
        # "Abort playback window and ourself"
        n312 = event-data() -> ()  [unwired: 1 in, 4 out]
        n313 = invoke class="VI" method="FP.Close"(reference=w490) -> (reference out=w489:refnum<vi>)  [unwired: 2 in, 2 out]
        n314 = invoke class="VI" method="Abort VI"(reference=w489) -> (error out=w488:errorcluster)  [unwired: 2 in, 2 out]
        n315 = invoke class="VI" method="Abort VI"(error in=w488) -> ()  [unwired: 2 in, 3 out]
      }
      event User Event {
        n316 = event-data() -> ("IDs"=w497:cluster{"RPC field ID":u16, "Unique ID":u16}, "String"=w496:string)  [unwired: 1 in]
        n317 = Bundle("IDs"=w497, "String"=w496) -> (w495:T14)  [unwired: 1 in]
        n318 = call <vilib>:"Retrieve RPC Response.vi"("RPC Response"=w495) -> ("Output"=w493:string[][])  [unwired: 10 in]
        n319 = Build Array (concatenate)(w491, w493) -> (w492:string[][])
        n320 = local write "Command Params"(w492) -> ()
        n321 = local write "Cmd Status"("" ("Cmd Status")) -> ()
      }
      event "Tree": Double Click {
        n322 = event-data() -> ("PlatMods"=w501:T30, "Tag"=w500:string)  [unwired: 1 in]
        n323 = Unbundle(w501) -> ("Shift"=w499:bool)  [unwired: 4 out]
        n324 = Not(x=w499) -> (.not. x?=w498:bool)
        n325 = call <vilib>:"NT Update Persistence.vi"("Persistence"=w498, "Name"=w500) -> ()  [unwired: 9 in, 1 out]
      }
    }
  }
  n326 = while {
    tunnel: w64 -> [w504]
    i -> [w507]
    stop <- FALSE stop-if-true
    n327 = Wait (ms)(milliseconds to wait=u32 100) -> ()  [unwired: 1 out]
    n328 = case shown="\"Playback\"" "Rec Mode" {
      tunnel: w507 -> [_ _ w522]
      tunnel: [u32 2829099 ("Base Color") u32 11141120 ("Target Color") w511] -> w503
      frame "Stop", Default {
        # "Reset the color, extra updates don't cost much"
      }
      frame "Record" {
      }
      frame "Playback" {
        # "Playback"
        n329 = Quotient & Remainder(x=w522, y=u32 50 ("milliseconds to wait")) -> (x-y*floor(x/y)=w518:u32)  [unwired: 1 out]
        n330 = Divide(x=w518, y=u32 50 ("milliseconds to wait")) -> (x/y=w515:dbl)
        n331 = Multiply(x=6.283185307179586, y=w515) -> (x*y=w520:dbl)
        n332 = Sine(x=w520) -> (sin(x)=w519:dbl)
        n333 = Absolute Value(x=w519) -> (abs(x)=w512:dbl)
        n334 = call "Interpolate RGB Color.vi"("Proportion"=w512, "Target Color"=u32 30976, "Base Color"=u32 2829099) -> ("Result Color"=w511:u32)  [unwired: 8 in]
      }
    }
    n335 = property class="Pane"(reference=w504, "PaneColor"=w503) -> ()  [unwired: 1 in, 2 out]
  }
  n336 = local write "Dashboard Tab"(T2."Drive" ("Dashboard Tab")) -> ()
  n337 = property on="On/Off" class="Bool (strict)"("Visible"=w34) -> ()  [unwired: 2 in, 2 out]
  n338 = property on="Motor" class="Clust (strict)"("Visible"=w34) -> ()  [unwired: 2 in, 2 out]
  n339 = property on="Progress" class="Clust (strict)"("Visible"=w34) -> ()  [unwired: 2 in, 2 out]
  n340 = property on="Test Ring" class="Ring (strict)"("Visible"=w34) -> ()  [unwired: 2 in, 2 out]
  n341 = property on="Rev/Fwd" class="Clust (strict)"("Visible"=w34) -> ()  [unwired: 2 in, 2 out]
  n342 = local write "Command Selection"(u16 0 ("milliseconds to wait")) -> ()
  n343 = local write "Command Params"(string[][] [] ("Command Params")) -> ()
  n344 = global write "WPI_DashboardLogging Global.vi" "Recording"(w58) -> ()
  n345 = local write "Rec Mode"(w58) -> ()
  n346 = while {
    tunnel: u16 1741 ("timeout ms (25000)") -> [w524]
    stop <- FALSE stop-if-true
    n347 = TCP Create Listener(10:w524) -> (0:w523:errorcluster, 3:w525:refnum<k5>)  [unwired: 4 in, 1 out]
    n348 = case shown="No Error" w523 {
      selector: w523 -> [w527 _]
      tunnel: w525 -> [w528 _]
      frame No Error {
        n349 = while {
          tunnel: w528 -> [w531]
          tunnel: w527 -> [w530]
          stop <- FALSE stop-if-true
          n350 = TCP Wait On Listener(8:w530, 11:w531) -> (0:w532:errorcluster, 4:w533:refnum<k5>)  [unwired: 2 in, 3 out]
          n351 = local write "TCP"(w533) -> ()
          n352 = case shown="No Error" w532 {
            frame No Error {
            }
            frame Error {
              n353 = Wait (ms)(milliseconds to wait=u32 1000) -> ()  [unwired: 1 out]
            }
          }
        }
      }
      frame Error {
        n354 = Wait (ms)(milliseconds to wait=u32 1000) -> ()  [unwired: 1 out]
      }
    }
  }
  n355 = call <vilib>:"NT Write String.vi"("String"="Select Auto", "Name"="Auto Selector") -> ()  [unwired: 9 in, 1 out]
